vi "Start_Stop_Timer.vi"(8 "error in (no error)":errorcluster, 10 "System data":T1, 11 "User Event in":refnum<user-event>) -> (0 "error out":errorcluster)   [LabVIEW 2023]
uses:
  Controls/System_Data.ctl
  Controls/Wash Options.ctl
  Controls/State.ctl
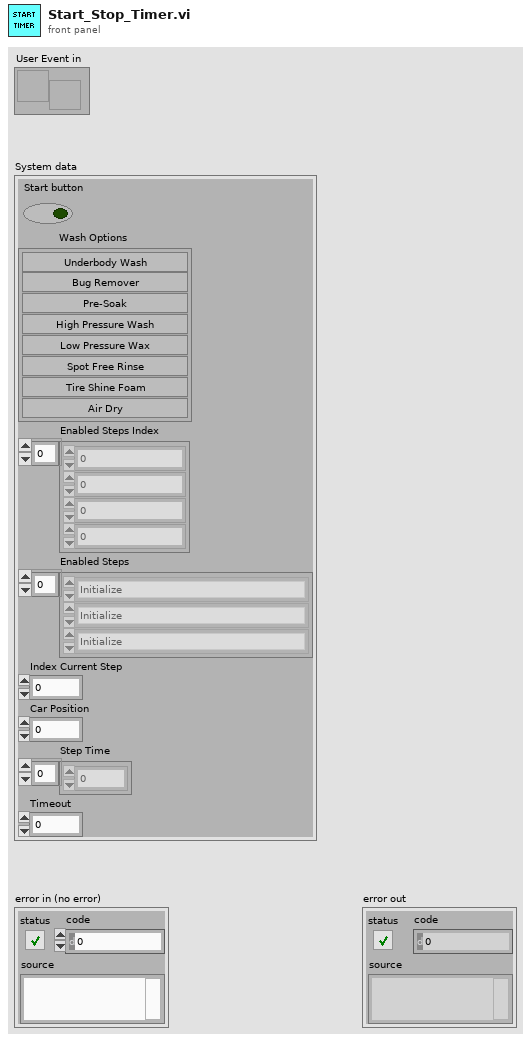
[diagram p1: front panel]
types:
  T1 = typedef "System_Data.ctl" = cluster{"Start button":bool, "Wash Options":T2, "Enabled Steps Index":i32[], "Enabled Steps ":T3[], "Index Current Step":i32, "Car Position":u8, "Step Time":dbl[], "Timeout":i32}
  T2 = typedef "Wash Options.ctl" = cluster{"Underbody Wash":bool, "Bug Remover":bool, "Pre-Soak":bool, "High Pressure Wash":bool, "Low Pressure Wax":bool, "Spot Free Rinse":bool, "Tire Shine Foam":bool, "Air Dry":bool}
  T3 = typedef "State.ctl" = enum16{"Initialize", "Wait for Something", "Step Completed", "Save Wash Options", "Start Process", "Car Position", "Order Steps to follow", "Underbody Wash", "Bug Remover", "Pre-Soak", "High Pressure Wash", "Low Pressure Wax", "Spot Free Rinse", "Tire Shine Foam", "Air Dry", "Vehicle out of position", "Process Complete", "Stop Application"}
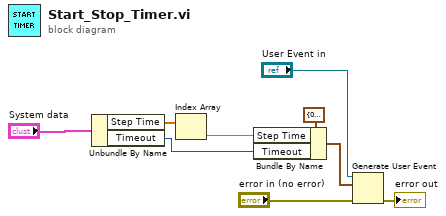
[diagram p0: block diagram]
diagram:
  n1 = Unbundle By Name("System data") -> ("Step Time"=w9:dbl[], "Timeout"=w1:i32)
  n2 = Index Array(array=w9) -> (element=w2:dbl)  [unwired: 1 in]
  n3 = Bundle By Name(cluster=cluster{"Step Time":dbl, "Timeout":i32} {"Step Time"=0.0, "Timeout"=0} ("event data"), "Step Time"=w2, "Timeout"=w1) -> (w3:cluster{"Step Time":dbl, "Timeout":i32})
  n4 = Generate User Event(user event="User Event in", event data cluster=w3, error in="error in (no error)") -> (error out=→"error out":errorcluster)  [unwired: 1 in, 1 out]
